vi "PDF_Interface_PDF Protokoll EPA1065_376 Chiller.vi"(8 "error in (no error)":errorcluster caption="Fehler (Eingang, kein Fehler)", 10 "ResultPictures":T1, 11 "Save PDF File Path":path) -> (0 "error out":errorcluster caption="Fehler (Ausgang)")   [LabVIEW 2020, in "EPA 1065.lvlib" / "Chiller NO2 1065-376.lvlib"]
uses:
  Chiller NO2 1065-376.lvlib
  T90 1065-308/Ergebnis.ctl
  PDF_Interface/PDF Interface Helper/PDFResultPictures.ctl
  Sprachverwaltung/FGV Aktion Tabelle zerlegen.ctl
  Seiten/FT-IR/FGV FT-IR Aktionen.ctl
  Seiten/System Einstellungen V2/Aktioen FGV System Konstanten.ctl
  Aktion FGV Chiller Test.ctl
  PDF_Interface/PDF Protokoll Standard Kopf Optionen.ctl
  Visualisierungs Elemente/Auswahlfeld.ctl
  PDF_Interface/PDF Protokoll Standard Kopf Gasflasche Auswahl.ctl
  <vilib>/Simplicity AI/SAI_PDF_API/Classes/Context/Controls/SAI_PDF_PDF Details.ctl
  PDF_Interface/PDF Interface Helper/PDFContentType.ctl
  PDF_Interface/PDF Interface Helper/PDFTableContentType.ctl
  PDF_Interface/PDF Interface Helper/PDFResults.ctl
  PDF_Interface/PDF Interface Helper/PDFCommentPosition.ctl
  PDF_Interface/PDF Interface Helper/PDFPageBreak.ctl
  PDF_Interface/PDF Interface Helper/PDFTablePictures.ctl
  PDF_Interface/PDF Interface Helper/PDFBemerkung.ctl
  <vilib>/Simplicity AI/SAI_PDF_API/Classes/Context/Controls/SAI_PDF_Text Align.ctl
  <vilib>/Simplicity AI/SAI_PDF_API/Classes/Context/Controls/SAI_PDF_Font.ctl
  <vilib>/Simplicity AI/SAI_PDF_API/Classes/Context/Controls/SAI_PDF_Font Encoding.ctl
  Allgemein/allgemeine Sub-VIs.lvlib
  Seiten/FT-IR/FT-IR.lvlib
  Seiten/System Einstellungen V2/System Einstellungen V2.lvlib
  PDF_Interface/PDF Interface.lvlib
  <vilib>/Simplicity AI/SAI_PDF_API/Classes/Context/Context.lvclass
  PDF_Interface/PDF Interface Helper/PDF Interface Helper.lvlib
  Sprachverwaltung/Sprachverwaltung.lvlib
  Linearisierung V2/Protokoll/Protokoll.lvlib
  T90 1065-308/T90 Test 1065-308.lvlib
panel:
  out "H2O":string caption="%"
  out "xNOxmeas":string caption="ppm"
  out "Ergebnis 1":T2
  out "xNOxmeas_dry":string caption="ppm"
  out "xNOxRef":string caption="ppm"
  out "Expiry Date":string caption="Expiry Date:"
  out "Versa Serial number:":string caption="Serial number:"
  out "Anlage:":string caption="Measuring Device:"
  out "Methode (Recipe):":string
  out "Date & Time:":string
  out "Accuracy:":string
  out "Gas Bottle Nr.:":string
  out "Ergebnis:":string caption="Result:"
  out "Konzentration:":string caption="Setpoint:"
  out "Komponente:":string caption="Component:"
  out "Bearbeiter:":string caption="Operator:"
  out "Serial number:":string
  out "Messgerät:":string caption="Analyzer:"
  # "Chiller Test EPA § 1065.376"
  # "xNOxmeas_dry ="
  # "/"
  # "(1-"
  # "/ 100)"
  # "x 0.95"
  # "<"
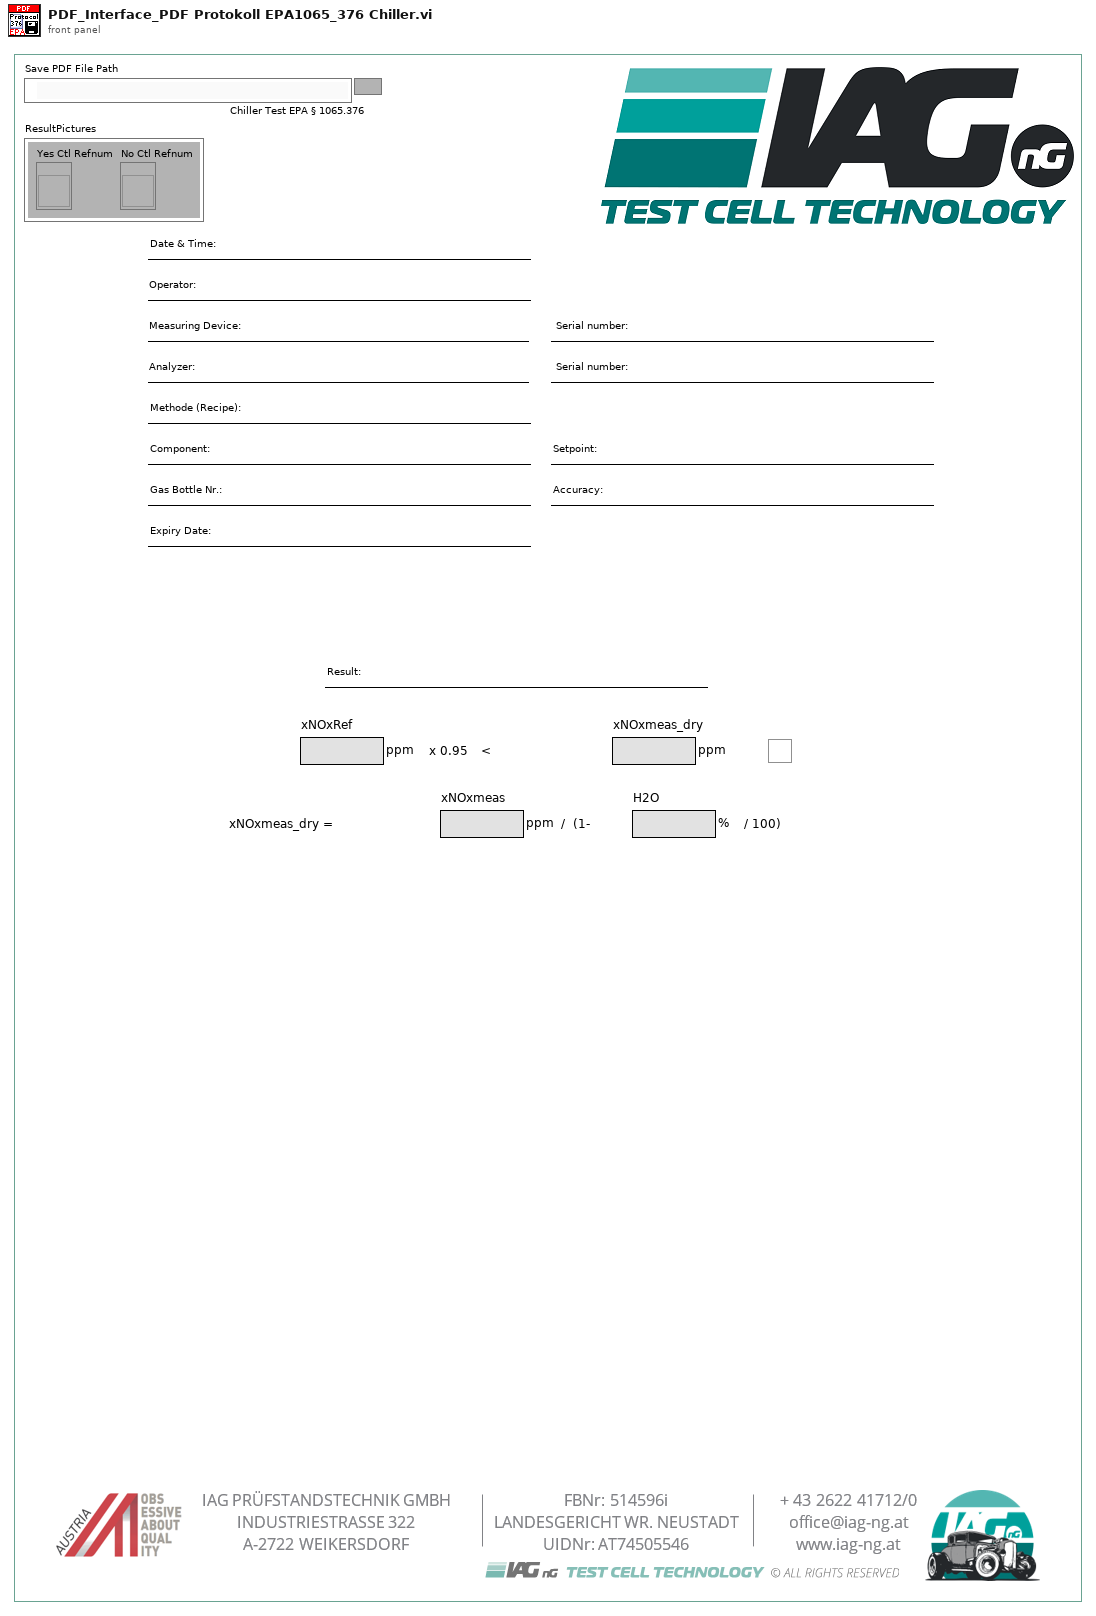
[diagram p1: front panel]
types:
  T1 = typedef "PDF Interface.lvlib/PDF Interface Helper.lvlib/PDFResultPictures.ctl" = cluster{"Yes Ctl Refnum":refnum<vi>, "No Ctl Refnum":refnum<vi>}
  T2 = typedef "EPA 1065.lvlib/T90 Test 1065-308.lvlib/Ergebnis.ctl" = bool
  T3 = typedef "Sprachverwaltung.lvlib/FGV Aktion Tabelle zerlegen.ctl" = enum16{"laden", "vereinzeln", "speichern"}
  T4 = typedef "PDF Interface.lvlib/PDF Protokoll Standard Kopf Gasflasche Auswahl.ctl" = cluster{"Gasflaschen Name":string, "Gasflaschen Nummer":string, "Gasnummer Index":i32}
  T5 = typedef "Auswahlfeld.ctl" = u16
  T6 = typedef "PDF Interface.lvlib/PDF Protokoll Standard Kopf Optionen.ctl" = cluster{"Analysator":bool, "FT-IR Rezept":bool, "Gasteiler":bool, "Gas Komponente":bool, "Gas Flasche":bool, "LIN Protokoll":bool, "Operator":bool}
  T7 = typedef "EPA 1065.lvlib/Chiller NO2 1065-376.lvlib/Aktion FGV Chiller Test.ctl" = enum16{"lesen", "Konfig Daten", "Messdaten", "Resultat", "Daten löschen", "PDF einstellen", "laden", "speichern"}
  T8 = typedef "System Einstellungen V2.lvlib/Aktioen FGV System Konstanten.ctl" = enum16{"lesen", "laden", "speichern", "Sprache"}
  T9 = typedef "FT-IR.lvlib/FGV FT-IR Aktionen.ctl" = enum16{"lesen", "NOG setzen", "NOS setzen", "Initialisieren", "speichern", "ALLES setzen", "FT-IR Spektrum loggen", "Komm Stoppen", "Spektrum LogKonfig"}
  T10 = typedef "PDF Interface.lvlib/PDF Interface Helper.lvlib/PDFResults.ctl" = cluster{"Results":cluster{"Result Text":string, "Result":bool}[], "ResultPictures":T1, "use Pictures":bool, "Image Scale (%)":sgl, "Autoscale? (T)":bool, "Horizontal Align":i32, "Position":i32}
  T11 = typedef "PDF Interface.lvlib/PDF Interface Helper.lvlib/PDFBemerkung.ctl" = cluster{"Bemerkung Text":string, "Align (Left)":T12, "Add Line Feeds (F:No)":bool, "Font":T13}
  T12 = typedef "SAI_PDF_Toolkit.lvlib/Context.lvclass/SAI_PDF_Text Align.ctl" = i32
  T13 = typedef "SAI_PDF_Toolkit.lvlib/Context.lvclass/SAI_PDF_Font.ctl" = cluster{"Font":string, "Size":i32, "Colour":u32, "Bold":bool, "Italic":bool, "Underline":bool, "Strikethrough":bool, "Font Encoding":T14}
  T14 = typedef "SAI_PDF_Toolkit.lvlib/Context.lvclass/SAI_PDF_Font Encoding.ctl" = enum16{"Cp1252, WinANSI", "IdentityH", "IdentityV", "Cp1250", "Cp1257", "MacRoman"}
  T15 = typedef "PDF Interface.lvlib/PDF Interface Helper.lvlib/PDFContentType.ctl" = cluster{"Titel":string, "Header Table":string[][], "Table Array":T16[], "Bemerkungen":T11[]}
  T16 = typedef "PDF Interface.lvlib/PDF Interface Helper.lvlib/PDFTableContentType.ctl" = cluster{"TableHeader":string[], "Table":string[][], "Relative Column Widths (%)":sgl[], "Results":T10, "PositionBemerkung":T17, "PageBreak":T18, "TablePictures":T19, "Horizontal Align":i32}
  T17 = typedef "PDF Interface.lvlib/PDF Interface Helper.lvlib/PDFCommentPosition.ctl" = enum16{"before", "after"}
  T18 = typedef "PDF Interface.lvlib/PDF Interface Helper.lvlib/PDFPageBreak.ctl" = enum16{"none", "before", "after", "after comment"}
  T19 = typedef "PDF Interface.lvlib/PDF Interface Helper.lvlib/PDFTablePictures.ctl" = cluster{"Ctl Refnum In":refnum<vi>[], "RowOrColumn":enum16{"Row", "Column"}, "IndexToInsert":u16, "Image Scale (%)":sgl[], "Autoscale? (T)":bool[], "Horizontal Align":i32}
  T20 = typedef "SAI_PDF_Toolkit.lvlib/Context.lvclass/SAI_PDF_PDF Details.ctl" = cluster{"Title":string, "Subject":string, "Keywords":string, "Author":string, "Creator":string}
  T21 = cluster{"Header Footer Text Cluster":cluster{"Header Text":string, "Footer Text":string, "Time":string, "Page Number":string}, "PDF Details":T20}
  T22 = cluster{"Modell":string, "ProjektNummer":string, "Software Version":string, "Seriennummer":string}
  T23 = typedef "EPA 1065.lvlib/Chiller NO2 1065-376.lvlib/Chiller Konfig Daten.ctl" = cluster{"Bearbeiter:":string, "Gasflaschen Nr.:":string, "Accuracy":dbl, "Sollwert":dbl, "Messgerät:":string, "Seriennummer:":string, "Pfad:":path, "Textname:":string, "Einheit":string, "Expiry Date":timestamp, "Water Concentration:":dbl, "Componente:":string}
  T24 = cluster{"Header Size":i32, "Column Ratio left":sgl[]}
  T25 = typedef "String - Ausgabefeld.ctl" = string
  T26 = typedef "EPA 1065.lvlib/Chiller NO2 1065-376.lvlib/Messdaten.ctl" = cluster{"xNOxRef":dbl, "xNOxmeas":dbl, "H2O":dbl, "xNOx_dry":dbl, "Bestanden":bool}
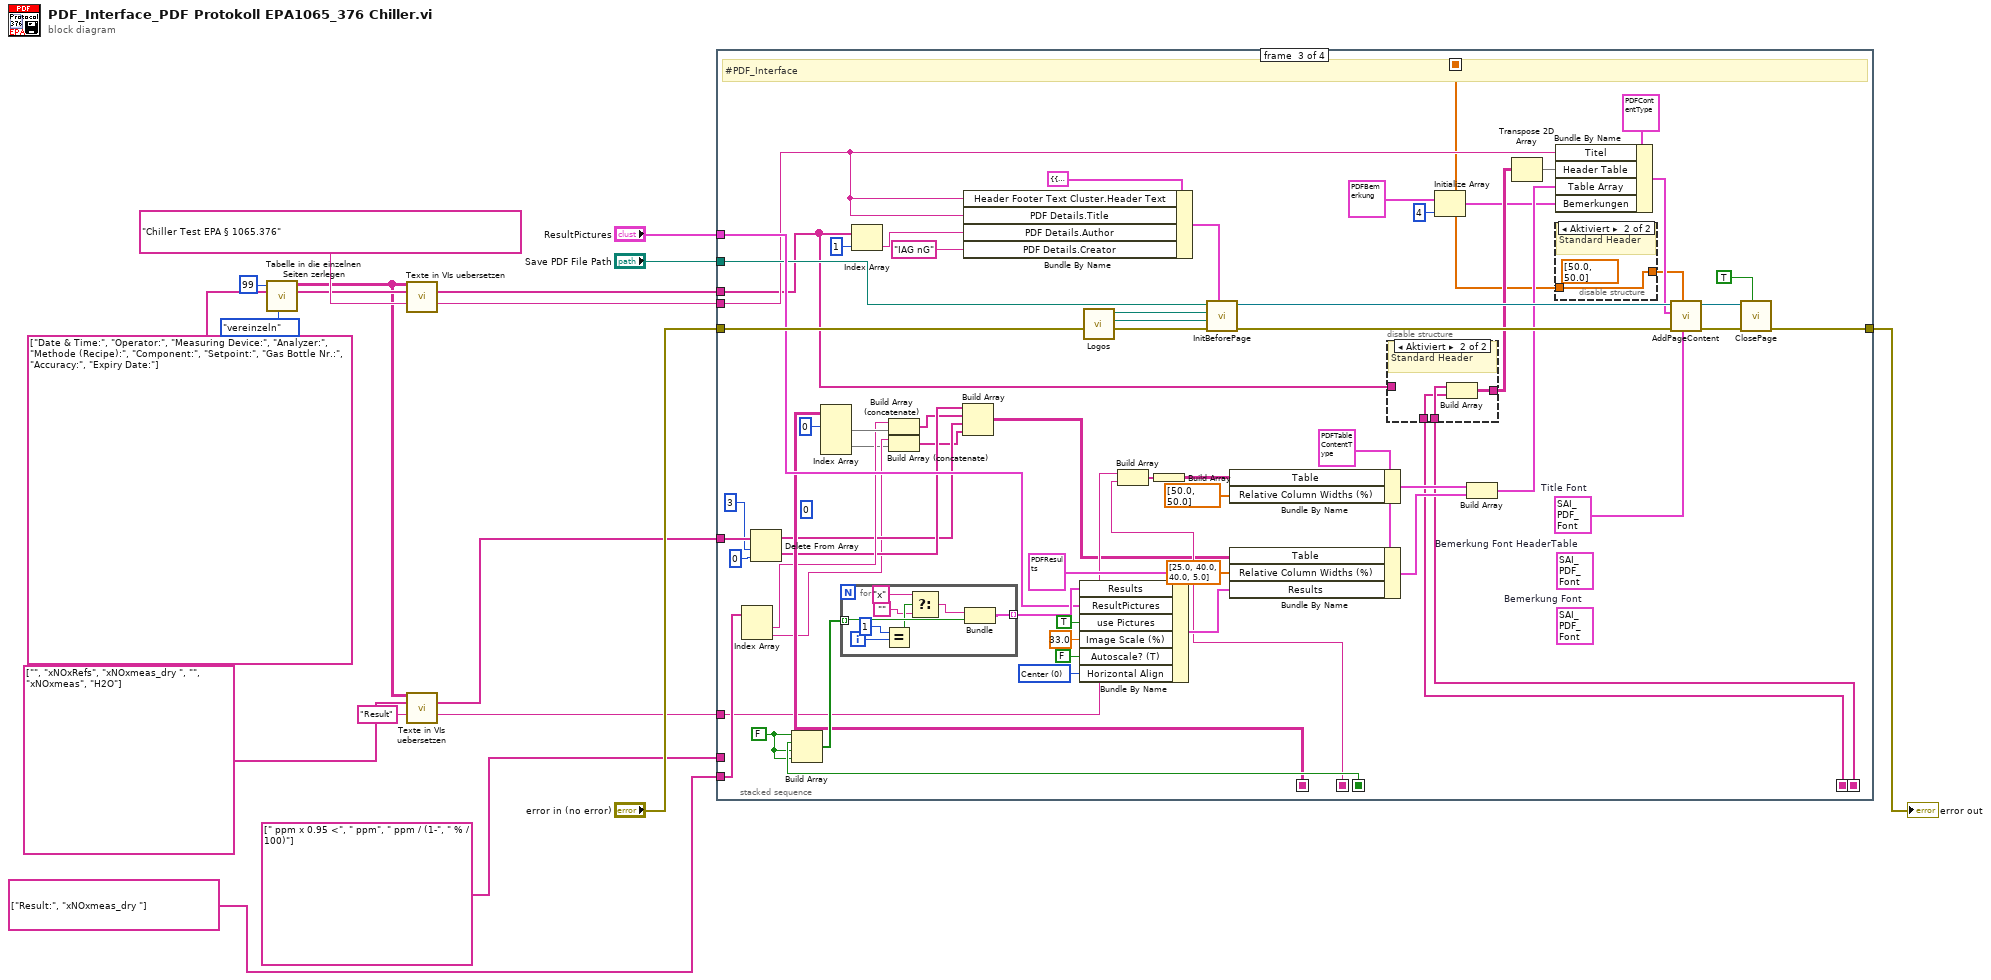
[diagram p0: block diagram]
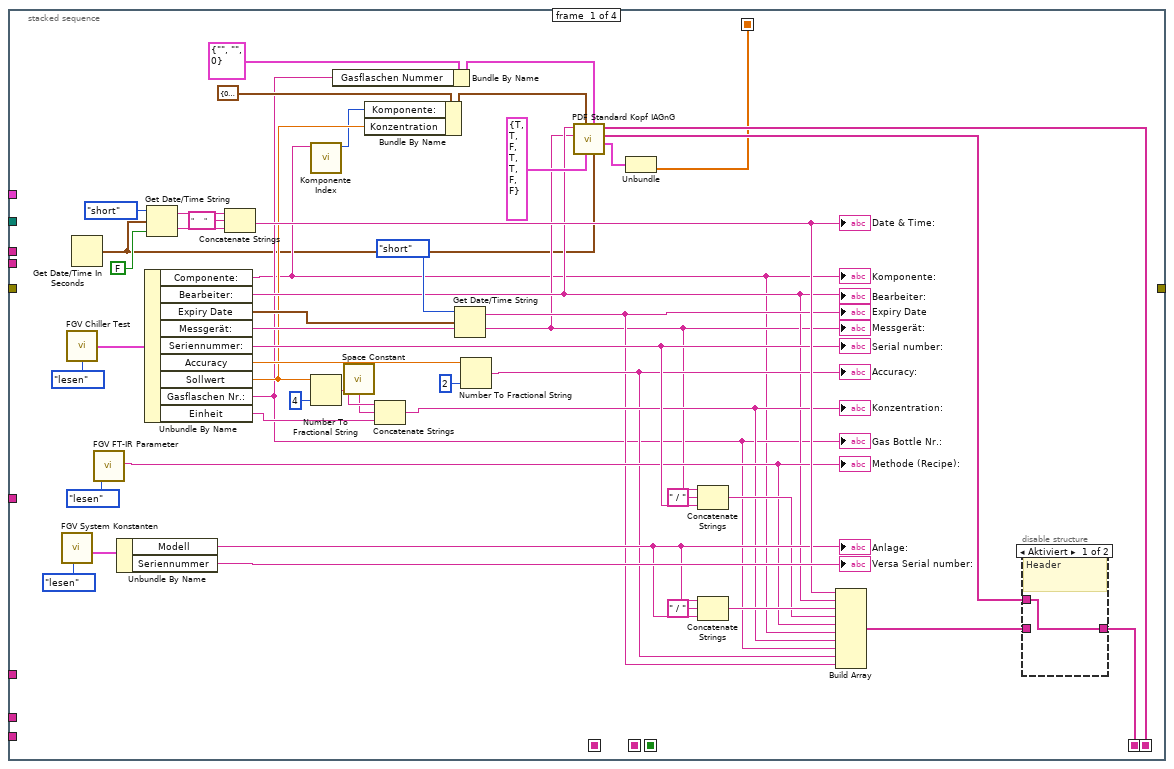
[diagram p2: hidden frame]
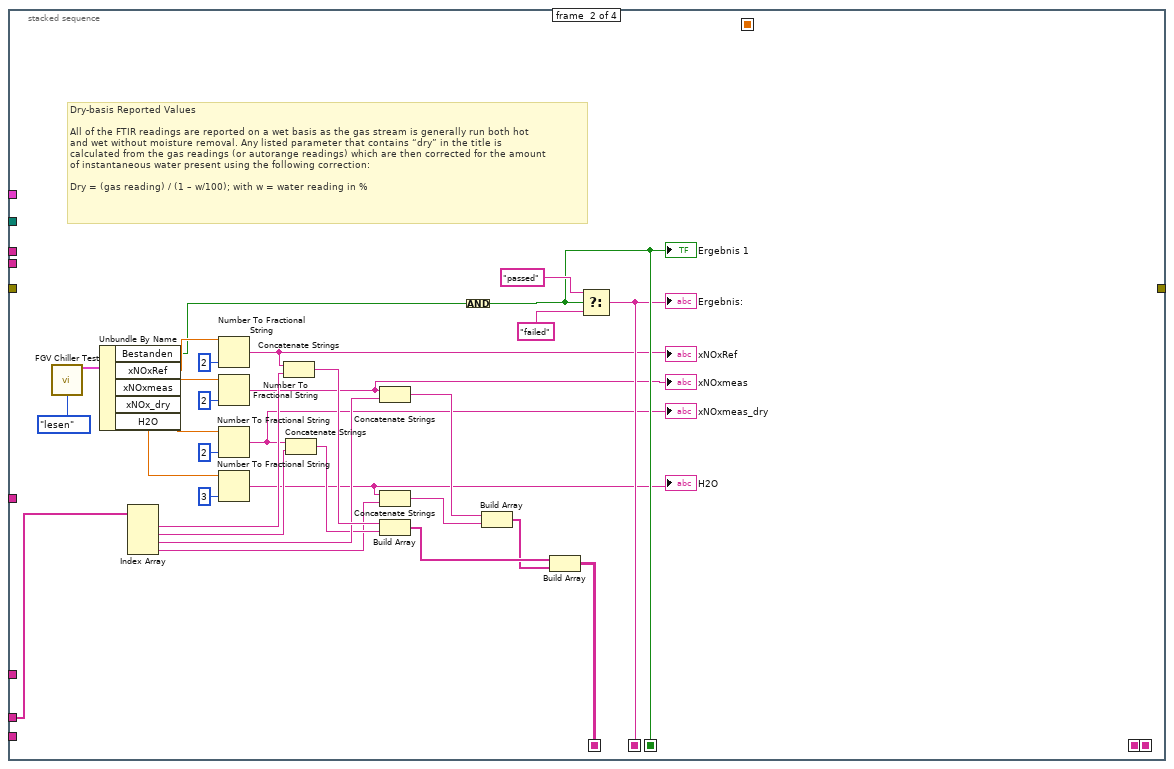
[diagram p4: hidden frame]
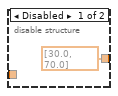
[diagram p5: hidden frame]
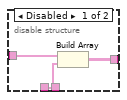
[diagram p6: hidden frame]
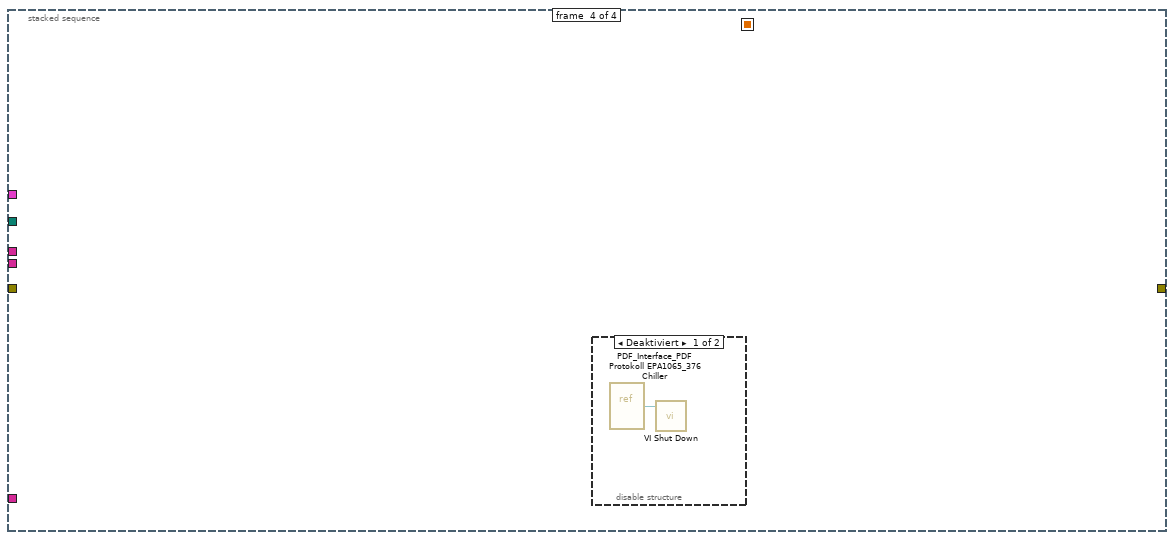
[diagram p7: hidden frame]
diagram:
  n1 = call "Tabelle in die einzelnen Seiten zerlegen.vi"("Aktion"=FGV_Aktion_Tabelle_zerlegen."vereinzeln", "Index (Seite)"=99) -> ("Sprachliste"=w8:string[][])  [unwired: 7 in, 2 out]
  n2 = call "Texte in VIs uebersetzen.vi"("Sprachliste"=w8, "String-Array zum Übersetzen"=string[] ["Date & Time:", "Operator:", "Measuring Device:", "Analyzer:", "Methode (Recipe):", "Component:", "Setpoint:", "Gas Bottle Nr.:", "Accuracy:", "Expiry Date:"], "String zum Übersetzen"="Chiller Test EPA § 1065.376") -> ("String-Array zum Übersetzen"=w5:string[], "String zum Übersetzen"=w6:string)  [unwired: 8 in, 3 out]
  n3 = call "Texte in VIs uebersetzen.vi"("Sprachliste"=w8, "String-Array zum Übersetzen"=string[] ["", "xNOxRefs", "xNOxmeas_dry ", "", "xNOxmeas", "H2O"], "String zum Übersetzen"="Result") -> ("String-Array zum Übersetzen"=w7:string[], "String zum Übersetzen"=w3:string)  [unwired: 8 in, 3 out]
  n4 = stacked-sequence {
    seq-local: [_ w85 _ _] -> [_ _ w126 _]
    seq-local: [w22 _ _ _] -> [_ _ w100 _]
    seq-local: [_ w84 _ _] -> [_ _ w121 _]
    seq-local: [_ w81 _ _] -> [_ _ w114 _]
    seq-local: [w21 _ _ _] -> [_ _ w101 _]
    seq-local: [w18 _ _ _] -> [_ _ w99 _]
    tunnel: "error in (no error)" -> [_ _ w131 _]
    tunnel: [_ _ w130 _] -> w16
    tunnel: "ResultPictures" -> [_ _ w129 _]
    tunnel: "Save PDF File Path" -> [_ _ w128 _]
    tunnel: w7 -> [_ _ w125 _]
    tunnel: w6 -> [_ _ w127 _]
    tunnel: w5 -> [_ _ w115 _]
    tunnel: w3 -> [_ _ w111 _]
    tunnel: string[] [" ppm x 0.95 <", " ppm", " ppm / (1-", " % / 100)"] -> [_ w80 _ _]
    tunnel: string[] ["Result:", "xNOxmeas_dry "] -> [_ _ w122 _]
    frame #0 {
      n5 = call "FGV System Konstanten.vi"("Aktionen"=Aktioen_FGV_System_Konstanten."lesen") -> ("Cluster out"=w52:T22)  [unwired: 6 in, 4 out]
      n6 = call "FGV Chiller Test.vi"("Aktion"=Aktion_FGV_Chiller_Test."lesen") -> ("Chiller Konfig Daten"=w50:T23)  [unwired: 11 in, 3 out]
      n7 = Get Date/Time In Seconds() -> (seconds since 1Jan1904=w20:timestamp)
      n8 = call "FGV FT-IR Parameter.vi"("Aktion"=FGV_FT-IR_Aktionen."lesen") -> ("Current Recipe"=w39:string)  [unwired: 11 in, 7 out]
      "Methode (Recipe):" <- w39
      n9 = Unbundle By Name(w52) -> ("Modell"=w45:string, "Seriennummer"=→"Versa Serial number:":string)
      "Anlage:" <- w45
      n10 = Unbundle By Name(w50) -> ("Componente:"=w26:string, "Bearbeiter:"=w34:string, "Expiry Date"=w48:timestamp, "Messgerät:"=w33:string, "Seriennummer:"=w43:string, "Accuracy"=w59:dbl, "Sollwert"=w30:dbl, "Gasflaschen Nr.:"=w27:string, "Einheit"=w54:string)
      "Gas Bottle Nr.:" <- w27
      "Messgerät:" <- w33
      "Bearbeiter:" <- w34
      "Serial number:" <- w43
      "Komponente:" <- w26
      n11 = Get Date/Time String(date format (0)=enum16{"short", "long", "abbreviated"}."short" ("Datumsformat (0)"), seconds (now)=w20, want seconds? (F)=FALSE ("Angabe von Sekunden? (F)")) -> (date string=w65:string, time string=w64:string)
      n12 = Concatenate Strings(w65, "     " ("String"), w64) -> (w46:string)
      "Date & Time:" <- w46
      n13 = call "Komponente Index.vi"("Komponente"=w26) -> ("Index in Gasliste"=w25:i32)  [unwired: 10 in]
      n14 = Number To Fractional String(number=w30, precision (6)=i16 4 ("Genauigkeit (6)")) -> (F-format string=w56:string)  [unwired: 2 in]
      n15 = Bundle By Name(cluster=T4 {"Gasflaschen Name"="", "Gasflaschen Nummer"="", "Gasnummer Index"=0} ("Gaschflasche Cluster"), "Gasflaschen Nummer"=w27) -> (w28:T4)
      n16 = call <vilib>:"Space Constant.vi"() -> ("String"=w55:string)
      n17 = Bundle By Name(cluster=cluster{"Komponente:":T5, "Konzentration":dbl} {"Komponente:"=0, "Konzentration"=0.0} ("Gas Komponente"), "Komponente:"=w25, "Konzentration"=w30) -> (w31:cluster{"Komponente:":T5, "Konzentration":dbl})
      n18 = Concatenate Strings(w56, w55, w54) -> (w38:string)
      "Konzentration:" <- w38
      n19 = Get Date/Time String(date format (0)=enum16{"short", "long", "abbreviated"}."short" ("Datumsformat (0)"), seconds (now)=w48) -> (date string=w36:string)  [unwired: 1 in, 1 out]
      "Expiry Date" <- w36
      n20 = Number To Fractional String(number=w59, precision (6)=i16 2 ("Genauigkeit (6)")) -> (F-format string=w37:string)  [unwired: 2 in]
      "Accuracy:" <- w37
      n21 = call "PDF Standard Kopf IAGnG.vi"("Zeitstempel"=w20, "Gaschflasche Cluster"=w28, "Oprtionen Cluster"=T6 {"Analysator"=TRUE, "FT-IR Rezept"=TRUE, "Gasteiler"=FALSE, "Gas Komponente"=TRUE, "Gas Flasche"=TRUE, "LIN Protokoll"=FALSE, "Operator"=FALSE}, "Gas Komponente"=w31, "Analysator"=w33, "Bearbeiter/in"=w34) -> ("Size Cluster"=w19:T24, "Header Values"=w24:T25[], "Header Labels"=w21:string[])  [unwired: 2 in, 1 out]
      n22 = Unbundle(w19) -> ("Column Ratio left"=w18:sgl[])  [unwired: 1 out]
      n23 = Concatenate Strings(w33, " / " ("String"), w43) -> (w40:string)
      n24 = Concatenate Strings(w45, " / " ("String"), w45) -> (w41:string)
      n25 = Build Array(w46, w34, w41, w40, w39, w26, w38, w27, w37, w36) -> (w23:string[])
      n26 = disable-structure shown="Aktiviert" {
        disable-tunnel: w24 -> [w66 _]
        disable-tunnel: w23 -> [_ w67]
        disable-tunnel: [w66 w67] -> w22
        frame Enabled {
          # "Standard Header"
        }
        frame Disabled {
        }
      }
    }
    frame #1 {
      # "Dry-basis Reported Values\n\nAll of the FTIR readings are reported on a wet basis as the gas stream is generally run both hot\nand wet without moisture removal. Any listed parameter that contains “dry” in the title is\ncalculated from the gas readings (or autorange readings) which are then corrected for the amount\nof instantaneous water present using the following correction:\n\nDry = (gas reading) / (1 – w/100); with w = water reading in %"
      n27 = call "FGV Chiller Test.vi"("Aktion"=Aktion_FGV_Chiller_Test."lesen") -> ("Daten"=w91:T26)  [unwired: 11 in, 3 out]
      n28 = Unbundle By Name(w91) -> ("Bestanden"=w87:bool, "xNOxRef"=w90:dbl, "xNOxmeas"=w89:dbl, "xNOx_dry"=w88:dbl, "H2O"=w86:dbl)
      n29 = Index Array(array=w80) -> (element #1=w79:string, element #2=w76:string, element #3=w75:string, element #4=w69:string)  [unwired: 4 in]
      n30 = Number To Fractional String(number=w90, precision (6)=i16 2 ("Genauigkeit (6)")) -> (F-format string=w78:string)  [unwired: 2 in]
      "xNOxRef" <- w78
      n31 = Number To Fractional String(number=w89, precision (6)=i16 2 ("Genauigkeit (6)")) -> (F-format string=w74:string)  [unwired: 2 in]
      "xNOxmeas" <- w74
      n32 = Number To Fractional String(number=w88, precision (6)=i16 2 ("Genauigkeit (6)")) -> (F-format string=w72:string)  [unwired: 2 in]
      "xNOxmeas_dry" <- w72
      n33 = Number To Fractional String(number=w86, precision (6)=i16 3 ("Genauigkeit (6)")) -> (F-format string=w70:string)  [unwired: 2 in]
      "H2O" <- w70
      n34 = Concatenate Strings(w78, w79) -> (w77:string)
      n35 = Concatenate Strings(w72, w76) -> (w71:string)
      n36 = Concatenate Strings(w74, w75) -> (w73:string)
      n37 = Concatenate Strings(w70, w69) -> (w68:string)
      n38 = Build Array(w77, w71) -> (w83:string[])
      n39 = Compound Arithmetic op=AND ("Mehrfacharithmetik")(w87) -> (w85:bool)
      "Ergebnis 1" <- w85
      n40 = Build Array(w73, w68) -> (w82:string[])
      n41 = Build Array(w83, w82) -> (w81:string[][])
      n42 = Select(t="passed", s=w85, f="failed") -> (s? t:f=w84:string)
      "Ergebnis:" <- w84
    }
    frame #2 {
      w102 = FALSE ("Element")
      (unwired) 0 ("Index (Zeile)")
      w132 = T12 0 items=["Center", "Justified", "Justified All", "Left", "Right"] ("Align (Left)")
      w116 = T16 {"TableHeader"=[], "Table"=[], "Relative Column Widths (%)"=[], "Results"={"Results"=[], "ResultPictures"={"Yes Ctl Refnum"=refnum, "No Ctl Refnum"=refnum}, "use Pictures"=FALSE, "Image Scale (%)"=0.0, "Autoscale? (T)"=FALSE, "Horizontal Align"=0, "Position"=0}, "PositionBemerkung"=enum."before", "PageBreak"=enum."none", "TablePictures"={"Ctl Refnum In"=[], "RowOrColumn"=enum."Row", "IndexToInsert"=0, "Image Scale (%)"=[], "Autoscale? (T)"=[], "Horizontal Align"=0}, "Horizontal Align"=0} ("Table Array")
      (unwired) T13 {"Font"="Arial", "Size"=12, "Colour"=16711680, "Bold"=TRUE, "Italic"=TRUE, "Underline"=FALSE, "Strikethrough"=FALSE, "Font Encoding"=enum."Cp1252, WinANSI"}  # Bemerkung Font HeaderTable
      (unwired) T13 {"Font"="Arial", "Size"=12, "Colour"=0, "Bold"=TRUE, "Italic"=TRUE, "Underline"=FALSE, "Strikethrough"=FALSE, "Font Encoding"=enum."Cp1252, WinANSI"}  # Bemerkung Font
      w145 = T13 {"Font"="Arial", "Size"=26, "Colour"=0, "Bold"=TRUE, "Italic"=FALSE, "Underline"=TRUE, "Strikethrough"=FALSE, "Font Encoding"=enum."Cp1252, WinANSI"}  # Title Font
      # "#PDF_Interface"
      n43 = Index Array(array=w122) -> (element #1=w109:string, element #2=w105:string)  [unwired: 2 in]
      n44 = Delete From Array(array=w125, length=3 ("Länge"), index=0 ("Länge")) -> (deleted portion=w108:string[], array with subset deleted=w106:string[])
      n45 = Build Array(w102, w126, w102, w102) -> (w140:bool[])
      n46 = Index Array(array=w114, index (row) #1=0 ("Index (Zeile)")) -> (element #1=w112:string[], element #2=w104:string[])  [unwired: 3 in]
      n47 = for {
        tunnel: w140 -> [w178] mode=indexing
        tunnel: [w179] -> w136 mode=indexing
        i -> [w175]
        n48 = Equal?(x=1 ("y"), y=w175) -> (x = y?=w173:bool)
        n49 = Select(t="x", s=w173, f="") -> (s? t:f=w176:string)
        n50 = Bundle(w176, "Element"=w178) -> (w179:cluster{string, "Element":bool})  [unwired: 1 in]
      }
      n51 = Index Array(array=w115, index=1 ("Index")) -> (element=w141:string)
      n52 = Build Array (concatenate)(w109, w112) -> (w107:string[])
      n53 = Build Array (concatenate)(w105, w104) -> (w103:string[])
      n54 = Build Array(w108, w107, w106, w103) -> (w110:string[][])
      n55 = Bundle By Name(cluster=T21 {"Header Footer Text Cluster"={"Header Text"="Protokoll XYZ", "Footer Text"="IAG nG", "Time"="<TIMESTAMP yyyy-MM-dd>", "Page Number"="Page <P> of <PT>"}, "PDF Details"={"Title"="Test PDF", "Subject"="Versa Tabasco", "Keywords"="", "Author"="RIW", "Creator"="IAG"}} ("Info"), "Header Footer Text Cluster.Header Text"=w127, "PDF Details.Title"=w127, "PDF Details.Author"=w141, "PDF Details.Creator"="IAG nG") -> (w154:T21)
      n56 = Bundle By Name(cluster=T10 {"Results"=[], "ResultPictures"={"Yes Ctl Refnum"=refnum, "No Ctl Refnum"=refnum}, "use Pictures"=FALSE, "Image Scale (%)"=100.0, "Autoscale? (T)"=TRUE, "Horizontal Align"=3, "Position"=0} ("Results"), "Results"=w136, "ResultPictures"=w129, "use Pictures"=TRUE, "Image Scale (%)"=sgl 33.0, "Autoscale? (T)"=FALSE, "Horizontal Align"=w132) -> (w137:T10)
      n57 = call "Logos.vi"() -> ("Footer Image File Path"=w162:path, "Header Image File Path"=w163:path)  [unwired: 8 in, 2 out]
      n58 = Build Array(w111, w121) -> (w120:string[])
      n59 = Build Array(w120) -> (w119:string[][])
      n60 = call "InitBeforePage.vi"("Info"=w154, "Fehler (Eingang, kein Fehler)"=w131, "Footer Image File Path"=w162, "Header Image File Path"=w163, "Path (Dialog if Empty)"=w128) -> ("Fehler (Ausgang)"=w161:errorcluster, "Context (Ausgang)"=w160:refnum<class "Context.lvclass">)  [unwired: 5 in]
      n61 = Bundle By Name(cluster=w116, "Table"=w119, "Relative Column Widths (%)"=sgl[] [50.0, 50.0]) -> (w117:T16)
      n62 = Bundle By Name(cluster=w116, "Table"=w110, "Relative Column Widths (%)"=sgl[] [25.0, 40.0, 40.0, 5.0], "Results"=w137) -> (w144:T16)
      n63 = disable-structure shown="Aktiviert" {
        disable-tunnel: [w168 w171] -> w152
        disable-tunnel: w115 -> [w166 _]
        disable-tunnel: w101 -> [_ w170]
        disable-tunnel: w100 -> [w167 w169]
        frame Disabled {
          n64 = Build Array(w166, w167) -> (w168:T25[][])
        }
        frame Enabled {
          # "Standard Header"
          n65 = Build Array(w170, w169) -> (w171:T25[][])
        }
      }
      n66 = Initialize Array(T11 {"Bemerkung Text"="", "Align (Left)"=0, "Add Line Feeds (F:No)"=FALSE, "Font"={"Font"="Arial", "Size"=10, "Colour"=0, "Bold"=FALSE, "Italic"=FALSE, "Underline"=FALSE, "Strikethrough"=FALSE, "Font Encoding"=enum."Cp1252, WinANSI"}} ("Bemerkung"), 4 ("Dimensionsgröße")) -> (w147:T11[])
      n67 = Build Array(w117, w144) -> (w151:T16[])
      n68 = Transpose 2D Array(2D array=w152) -> (transposed array=w148:T25[][])
      n69 = Bundle By Name(cluster=T15 {"Titel"="Test mit Graph und Results PDF", "Header Table"=[["Murks:", "4711"], ["HolyShit:", "0815"]], "Table Array"=[{"TableHeader"=["Soll\nppm/%", "Ist\nppm/%", "Fehler\n%", "Toleranz\n%", "Ergebnis"], "Table"=[["aaa", "bbb", "ccc", "ddd"], ["111", "222", "333", "444"], ["sss", "fff", "kkk", "xxx"], ["6.5", "11.13", "19.2", "4"], ["1111", "1212", "777", "888"]], "Relative Column Widths (%)"=[22.5, 22.5, 22.5, 22.5, 10.0], "Results"={"Results"=[], "ResultPictures"={"Yes Ctl Refnum"=refnum, "No Ctl Refnum"=refnum}, "use Pictures"=FALSE, "Image Scale (%)"=100.0, "Autoscale? (T)"=TRUE, "Horizontal Align"=3, "Position"=0}, "PositionBemerkung"=enum."after", "PageBreak"=enum."none", "TablePictures"={"Ctl Refnum In"=[], "RowOrColumn"=enum."Row", "IndexToInsert"=0, "Image Scale (%)"=[], "Autoscale? (T)"=[], "Horizontal Align"=3}, "Horizontal Align"=3}, {"TableHeader"=["Soll\nppm/%", "Ist\nppm/%", "Fehler\n%", "Toleranz\n%", "Ergebnis"], "Table"=[["aaa", "bbb", "ccc", "ddd"], ["111", "222", "333", "444"], ["sss", "fff", "kkk", "xxx"], ["6.5", "11.13", "19.2", "4"], ["1111", "1212", "777", "888"]], "Relative Column Widths (%)"=[22.5, 22.5, 22.5, 22.5, 10.0], "Results"={"Results"=[], "ResultPictures"={"Yes Ctl Refnum"=refnum, "No Ctl Refnum"=refnum}, "use Pictures"=FALSE, "Image Scale (%)"=100.0, "Autoscale? (T)"=TRUE, "Horizontal Align"=3, "Position"=0}, "PositionBemerkung"=enum."before", "PageBreak"=enum."before", "TablePictures"={"Ctl Refnum In"=[], "RowOrColumn"=enum."Row", "IndexToInsert"=0, "Image Scale (%)"=[], "Autoscale? (T)"=[], "Horizontal Align"=3}, "Horizontal Align"=3}, {"TableHeader"=["Soll\nppm/%", "Ist\nppm/%", "Fehler\n%", "Toleranz\n%", "Ergebnis"], "Table"=[["aaa", "bbb", "ccc", "ddd"], ["111", "222", "333", "444"], ["sss", "fff", "kkk", "xxx"], ["6.5", "11.13", "19.2", "4"], ["1111", "1212", "777", "888"]], "Relative Column Widths (%)"=[22.5, 22.5, 22.5, 22.5, 10.0], "Results"={"Results"=[], "ResultPictures"={"Yes Ctl Refnum"=refnum, "No Ctl Refnum"=refnum}, "use Pictures"=FALSE, "Image Scale (%)"=100.0, "Autoscale? (T)"=TRUE, "Horizontal Align"=3, "Position"=0}, "PositionBemerkung"=enum."before", "PageBreak"=enum."before", "TablePictures"={"Ctl Refnum In"=[], "RowOrColumn"=enum."Row", "IndexToInsert"=0, "Image Scale (%)"=[], "Autoscale? (T)"=[], "Horizontal Align"=3}, "Horizontal Align"=3}, {"TableHeader"=["Soll\nppm/%", "Ist\nppm/%", "Fehler\n%", "Toleranz\n%", "Ergebnis"], "Table"=[["aaa", "bbb", "ccc", "ddd"], ["111", "222", "333", "444"], ["sss", "fff", "kkk", "xxx"], ["6.5", "11.13", "19.2", "4"], ["1111", "1212", "777", "888"]], "Relative Column Widths (%)"=[22.5, 22.5, 22.5, 22.5, 10.0], "Results"={"Results"=[], "ResultPictures"={"Yes Ctl Refnum"=refnum, "No Ctl Refnum"=refnum}, "use Pictures"=FALSE, "Image Scale (%)"=100.0, "Autoscale? (T)"=TRUE, "Horizontal Align"=3, "Position"=0}, "PositionBemerkung"=enum."before", "PageBreak"=enum."before", "TablePictures"={"Ctl Refnum In"=[], "RowOrColumn"=enum."Row", "IndexToInsert"=0, "Image Scale (%)"=[], "Autoscale? (T)"=[], "Horizontal Align"=3}, "Horizontal Align"=3}, {"TableHeader"=["Soll\nppm/%", "Ist\nppm/%", "Fehler\n%", "Toleranz\n%", "Ergebnis"], "Table"=[["aaa", "bbb", "ccc", "ddd"], ["111", "222", "333", "444"], ["sss", "fff", "kkk", "xxx"], ["6.5", "11.13", "19.2", "4"], ["1111", "1212", "777", "888"]], "Relative Column Widths (%)"=[22.5, 22.5, 22.5, 22.5, 10.0], "Results"={"Results"=[], "ResultPictures"={"Yes Ctl Refnum"=refnum, "No Ctl Refnum"=refnum}, "use Pictures"=FALSE, "Image Scale (%)"=100.0, "Autoscale? (T)"=TRUE, "Horizontal Align"=3, "Position"=0}, "PositionBemerkung"=enum."before", "PageBreak"=enum."before", "TablePictures"={"Ctl Refnum In"=[], "RowOrColumn"=enum."Row", "IndexToInsert"=0, "Image Scale (%)"=[], "Autoscale? (T)"=[], "Horizontal Align"=3}, "Horizontal Align"=3}], "Bemerkungen"=[{"Bemerkung Text"="super geiles PDF", "Align (Left)"=0, "Add Line Feeds (F:No)"=TRUE, "Font"={"Font"="Arial", "Size"=10, "Colour"=0, "Bold"=FALSE, "Italic"=FALSE, "Underline"=FALSE, "Strikethrough"=FALSE, "Font Encoding"=enum."Cp1252, WinANSI"}}, {"Bemerkung Text"="", "Align (Left)"=0, "Add Line Feeds (F:No)"=FALSE, "Font"={"Font"="Arial", "Size"=10, "Colour"=0, "Bold"=FALSE, "Italic"=FALSE, "Underline"=FALSE, "Strikethrough"=FALSE, "Font Encoding"=enum."Cp1252, WinANSI"}}, {"Bemerkung Text"="Tabelle mit optionalen Ergebnissen", "Align (Left)"=3, "Add Line Feeds (F:No)"=FALSE, "Font"={"Font"="Arial", "Size"=10, "Colour"=0, "Bold"=FALSE, "Italic"=FALSE, "Underline"=FALSE, "Strikethrough"=FALSE, "Font Encoding"=enum."Cp1252, WinANSI"}}, {"Bemerkung Text"="Graph geht ab ... ", "Align (Left)"=0, "Add Line Feeds (F:No)"=FALSE, "Font"={"Font"="Arial", "Size"=10, "Colour"=0, "Bold"=FALSE, "Italic"=FALSE, "Underline"=FALSE, "Strikethrough"=FALSE, "Font Encoding"=enum."Cp1252, WinANSI"}}]} ("Content"), "Titel"=w127, "Header Table"=w148, "Table Array"=w151, "Bemerkungen"=w147) -> (w150:T15)
      n70 = disable-structure shown="Aktiviert" {
        disable-tunnel: [sgl[] [30.0, 70.0] ("Column Ratio left") w165] -> w149
        disable-tunnel: w99 -> [_ w165]
        frame Disabled {
        }
        frame Enabled {
          (unwired) sgl[] [50.0, 50.0] ("Column Ratio left")
          # "Standard Header"
        }
      }
      n71 = call "AddPageContent.vi"("Title Font"=w145, "Column Ratio left"=w149, "error in"=w161, "Content"=w150, "Context (Eingang)"=w160) -> ("error out"=w159:errorcluster, "Context (Ausgang)"=w158:refnum<class "Context.lvclass">)  [unwired: 5 in]
      n72 = call "ClosePage.vi"("popup viewer"=TRUE, "Fehler (Eingang, kein Fehler)"=w159, "Context (Eingang)"=w158) -> ("Fehler (Ausgang)"=w130:errorcluster)  [unwired: 8 in]
    }
    frame #3 {
      n73 = disable-structure shown="Deaktiviert" {
        frame Disabled {
          n74 = vi-ref "PDF_Interface_PDF Protokoll EPA1065_376 Chiller.vi"() -> (w180:refnum<vi>)
          n75 = call "VI Shut Down.vi"("VI Referenz"=w180) -> ()  [unwired: 11 in]
        }
        frame Enabled {
        }
      }
    }
  }
  "error out" <- w16
